vi "Hybrid Start Server.vi"() -> ()   [LabVIEW 2024]
doc: "This is a simple example of a server which exports VIs to be called from another machine. You may run both the client.llb and server.llb on the same machine without modifying the access list. If you wish to run the client on another machine that is not in your domain you will have to list the name of the client in the Machine Access List. \n\nThe VIs listed in the Exported VI list are exported by the server.\n\nTo run this example start this VI First, then start the client.llb on all machines you want to try as clients. If you change either of the above lists, you must restart this VI for the changes to take effect.\n\nClick the \"Stop\" button to quit. This will turn off the server, terminating all client connections, and restore the previous access lists to their original values."
panel:
  out "error out":errorcluster
  in  "stop":bool
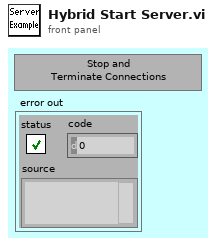
[diagram p1: front panel]
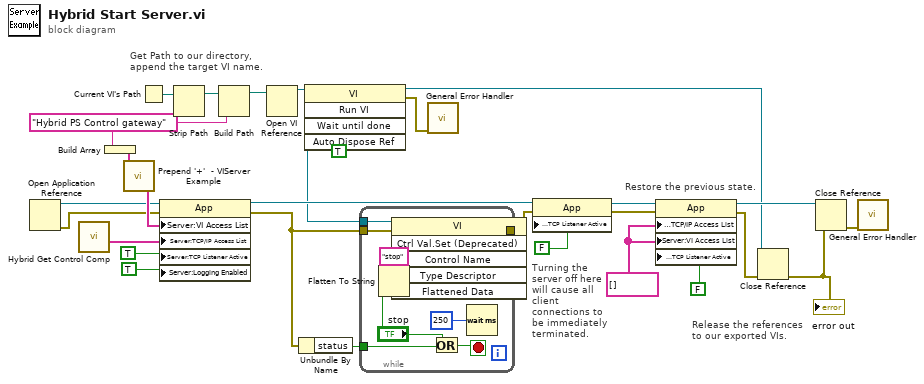
[diagram p0: block diagram]
diagram:
  w1 = string[] [] ("Server:TCP/IP Access List")
  w10 = "Hybrid PS Control gateway"
  # "Get Path to our directory,\nappend the target VI name."
  # "Turning the server off here will cause all client connections to be immediately\nterminated."
  # "Release the references\nto our exported VIs."
  # "Restore the previous state."
  n1 = Open Application Reference() -> (0:w2:errorcluster, 3:w3:refnum<vi>)  [unwired: 4 in]
  n2 = call "Hybrid Get Control Comp.vi"() -> ("Client 2"=w15:string[])
  n3 = Build Array(w10) -> (w11:string[])
  n4 = call "Prepend '+'  - VIServer Example.vi"("list in"=w11) -> ("list out"=w27:string[])
  n5 = Current VI's Path() -> (path=w14:path)
  n6 = property class="App"(reference=w3, error in=w2, "Server:VI Access List"=w27, "Server:TCP/IP Access List"=w15, "Server:TCP Listener Active"=TRUE ("Srvr.TCPActive"), "Server:Logging Enabled"=TRUE ("Srvr.LogEnabled")) -> (reference out=w19:refnum<vi>, error out=w7:errorcluster)
  n7 = Strip Path(path=w14) -> (stripped path=w12:path)  [unwired: 1 out]
  n8 = Build Path(base path=w12, name or relative path=w10) -> (appended path=w13:path)
  n9 = Open VI Reference(vi path=w13) -> (vi reference=w5:refnum<vi>)  [unwired: 5 in, 1 out]
  n10 = Unbundle By Name(w7) -> ("status"=w25:bool)
  n11 = invoke class="VI" method="Run VI"(reference=w5, "Wait until done"=TRUE) -> (reference out=w4:refnum<vi>, error out=w8:errorcluster)  [unwired: 3 in, 3 out]
  n12 = while {
    tunnel: [w29] -> w6
    tunnel: w5 -> [w33]
    tunnel: w7 -> [w34]
    tunnel: w25 -> [w36]
    stop <- w37 stop-if-true
    n13 = Flatten To String(anything="stop") -> (data string=w30:string, type string=w31:i16[])  [unwired: 3 in, 1 out]
    n14 = invoke class="VI" method="Ctrl Val.Set (Deprecated)"(reference=w33, error in=w34, "Control Name"="stop", "Type Descriptor"=w31, "Flattened Data"=w30) -> (error out=w29:errorcluster)  [unwired: 1 in, 5 out]
    n15 = Or(x="stop", y=w36) -> (x .or. y?=w37:bool)
    n16 = Wait (ms)(milliseconds to wait=u32 250) -> ()  [unwired: 1 out]
  }
  n17 = call <vilib>:"General Error Handler.vi"("error in (no error)"=w8) -> ()  [unwired: 10 in, 5 out]
  n18 = property class="App"(reference=w19, error in=w6, "Server:TCP Listener Active"=FALSE ("Srvr.TCPActive")) -> (reference out=w20:refnum<vi>, error out=w21:errorcluster)
  n19 = property class="App"(reference=w20, error in=w21, "Server:TCP/IP Access List"=w1, "Server:VI Access List"=w1, "Server:TCP Listener Active"=FALSE) -> (reference out=w28:refnum<vi>, error out=w24:errorcluster)
  n20 = Close Reference(reference=w4, error in (no error)=w24) -> (error out=w23:errorcluster)
  "error out" <- w23
  n21 = Close Reference(reference=w28, error in (no error)=w23) -> (error out=w22:errorcluster)
  n22 = call <vilib>:"General Error Handler.vi"("error in (no error)"=w22) -> ()  [unwired: 10 in, 5 out]
